vi "protect ui.vi"(10 "EVENT":refnum<user-event>, 11 "DVR":refnum<data-value>) -> ()   [LabVIEW 2013, in "protection settings.lvclass"]
uses:
  protection settings.lvclass
  VI modification.lvclass
  protection settings.lvclass/protection settings.ctl
panel:
  in  "password (opt)":string
  in  "Lock State":T1(ring)=enum."Locked (No Password)"
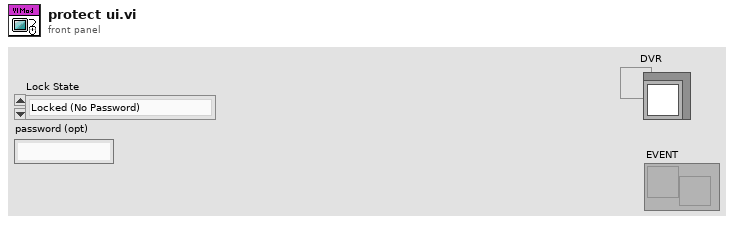
[diagram p1: front panel]
types:
  T1 = enum32{"invalid lock state", "Not Locked", "Locked (No Password)", "Password-protected"}
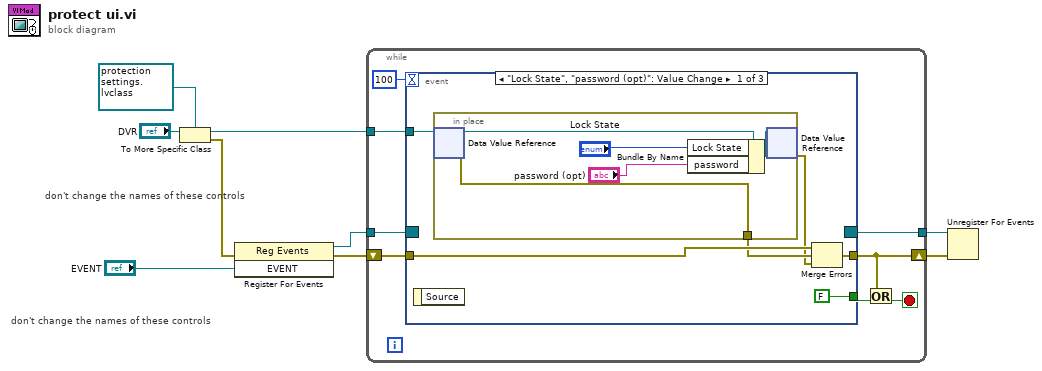
[diagram p0: block diagram]
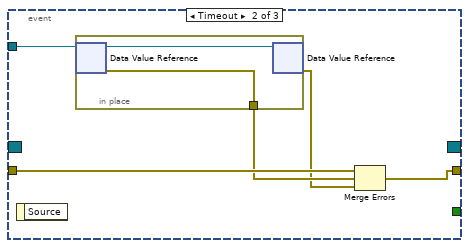
[diagram p2: hidden frame]
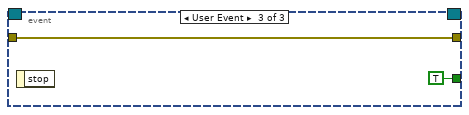
[diagram p3: hidden frame]
diagram:
  # "don't change the names of these controls"
  # "don't change the names of these controls"
  n1 = To More Specific Class(target class=refnum<data-value> refnum, reference="DVR") -> (specific class reference=w3:refnum<data-value>, error out=w1:errorcluster)  [unwired: 1 in]
  n2 = register-events(error in=w1, "EVENT") -> (reference out=w7:refnum<event-registration>, error out=w8:errorcluster)  [unwired: 1 in]
  n3 = while {
    shift-right: [w10] -> w6
    shift-left: w8 -> [w14]
    tunnel: w7 -> [w17]
    tunnel: [w16] -> w5
    tunnel: w3 -> [w13]
    stop <- w11 stop-if-true
    n4 = event shown="[0] \"Lock State\", \"password (opt)\": Value Change" {
      selector: w17 -> [_ _ _]
      dyn-events: [_ _ _] -> w16
      timeout: 100 -> [_ _ _]
      tunnel: [FALSE _ TRUE] -> w15
      tunnel: [w21 w31 w37] -> w10
      tunnel: w14 -> [w23 w32 w37]
      tunnel: w13 -> [w22 w33 _]
      event "Lock State", "password (opt)": Value Change {
        n5 = event-data() -> ()  [unwired: 1 in, 1 out]
        n6 = in-place {
          in-place-border: [w26] -> w19
          n7 = in-place-dvr #1(w22) -> (w28:refnum<class "protection settings.lvclass">, w26:errorcluster)
          n8 = Bundle By Name(cluster=w28, "Lock State"="Lock State", "password"="password (opt)") -> (w27:refnum<class "protection settings.lvclass">)
          n9 = in-place-dvr #1(w27) -> (w18:errorcluster)  [unwired: 1 out]
        }
        n10 = Merge Errors(w23, w19, w18) -> (w21:errorcluster)
      }
      event Timeout {
        n11 = event-data() -> ()  [unwired: 1 in, 1 out]
        n12 = in-place {
          in-place-border: [w34] -> w30
          n13 = in-place-dvr #2(w33) -> (w35:refnum<class "protection settings.lvclass">, w34:errorcluster)
          n14 = in-place-dvr #2(w35) -> (w29:errorcluster)  [unwired: 1 out]
        }
        n15 = Merge Errors(w32, w30, w29) -> (w31:errorcluster)
      }
      event User Event {
        n16 = event-data() -> ()  [unwired: 1 in, 1 out]
      }
    }
    n17 = Or(x=w10, y=w15) -> (x .or. y?=w11:bool)
  }
  n18 = Unregister For Events(event registration refnum=w5, error in=w6) -> ()  [unwired: 1 out]
